vi "Capacitance_IS_Configure.vi"(0 "Semiconductor Module Context":T7, 1 "DCPower Pin":tag, 2 "Scope Pins":tag[](array[tag]), 3 "FGEN Pin":tag, 4 "SCOPE Parameters":T4={"min sample rate"=20000000.0, "min record length"=1000, "reference position"=5.0, "input impedance"=0, "maximum input frequency"=0.0, "vertical coupling"=1, "vertical range"=10.0, "vertical offset"=0.0, "NumRecords"=0} {"maximum input frequency" format="%.2f"; "input impedance" items=["1 mega ohm"=0, "50 ohms"=2]; "vertical offset" format="%.4f"; "vertical range" format="%.2f"; "vertical coupling" items=["AC", "DC", "Ground"]; "reference position" format="%#_13g"; "min sample rate" format="%^.2e"}, 5 "FGEN Parameters":T2 {"Trigger Mode" items=["Single", "Continuous", "Stepped", "Burst"]}, 6 "DCPower_Parameters":T6={"Output"=enum."DC Voltage", "Current_range"=0.0, "Current"=0.0, "Voltage_range"=0.0, "Voltage"=0.0, "Aperture_time"=0.0, "Source Delay"=0.0, "Sense"=1008} {"Source Delay" format="%.6p"; "Sense" items=["Local"=1008, "Remote"=1009]; "Aperture_time" format="%.6p"; "Current_range" format="%.6p"; "Current" format="%.6p"; "Voltage_range" format="%.6p"; "Voltage" format="%.6p"}) -> (14 "FFT Subset Parameters":T1, 19 "error out":errorcluster)   [LabVIEW 2023, in "Capacitance.lvlib"]
doc: "Configure DCPower, SCOPE and FGEN sessions for impedance spectroscopy measurement"
uses:
  Capacitance.lvlib
  <vilib>/NI_TestStand_SemiconductorModule/NI_TestStand_Semiconductor_Module.lvlibp/PinMap/General/SemiconductorModuleContext.ctl
  ResourceHandling/TypeDefs/RH_DCPower_Parameters.ctl
  ResourceHandling/TypeDefs/RH_SCOPE_Parameters.ctl
  <instrlib>/niScope/Controls/niScope vertical coupling.ctl
  ResourceHandling/TypeDefs/RH_FGEN_Parameters.ctl
  <instrlib>/niFgen/niFgen.llb/niFgen Trigger Mode.ctl
  <instrlib>/niFgen/niFgen.llb/niFgen_ctl Exported Signal Desination Values (ComboBox).ctl
  <instrlib>/niScope/Controls/niScope trigger source digital.ctl
  <vilib>/NI_TestStand_SemiconductorModule/NI_TestStand_Semiconductor_Module.lvlibp/PinMap/DC Power/PinToNIDCPowerSessions.vi
  <vilib>/NI_TestStand_SemiconductorModule/NI_TestStand_Semiconductor_Module.lvlibp/PinMap/Scope/PinsToNISCOPESession.vi
  <vilib>/NI_TestStand_SemiconductorModule/NI_TestStand_Semiconductor_Module.lvlibp/PinMap/FGEN/PinToNIFGenSession.vi
  <vilib>/NI_TestStand_SemiconductorModule/NI_TestStand_Semiconductor_Module.lvlibp
  ResourceHandling/ResourceHandling.lvlib
  Resonance/Resonance.lvlib
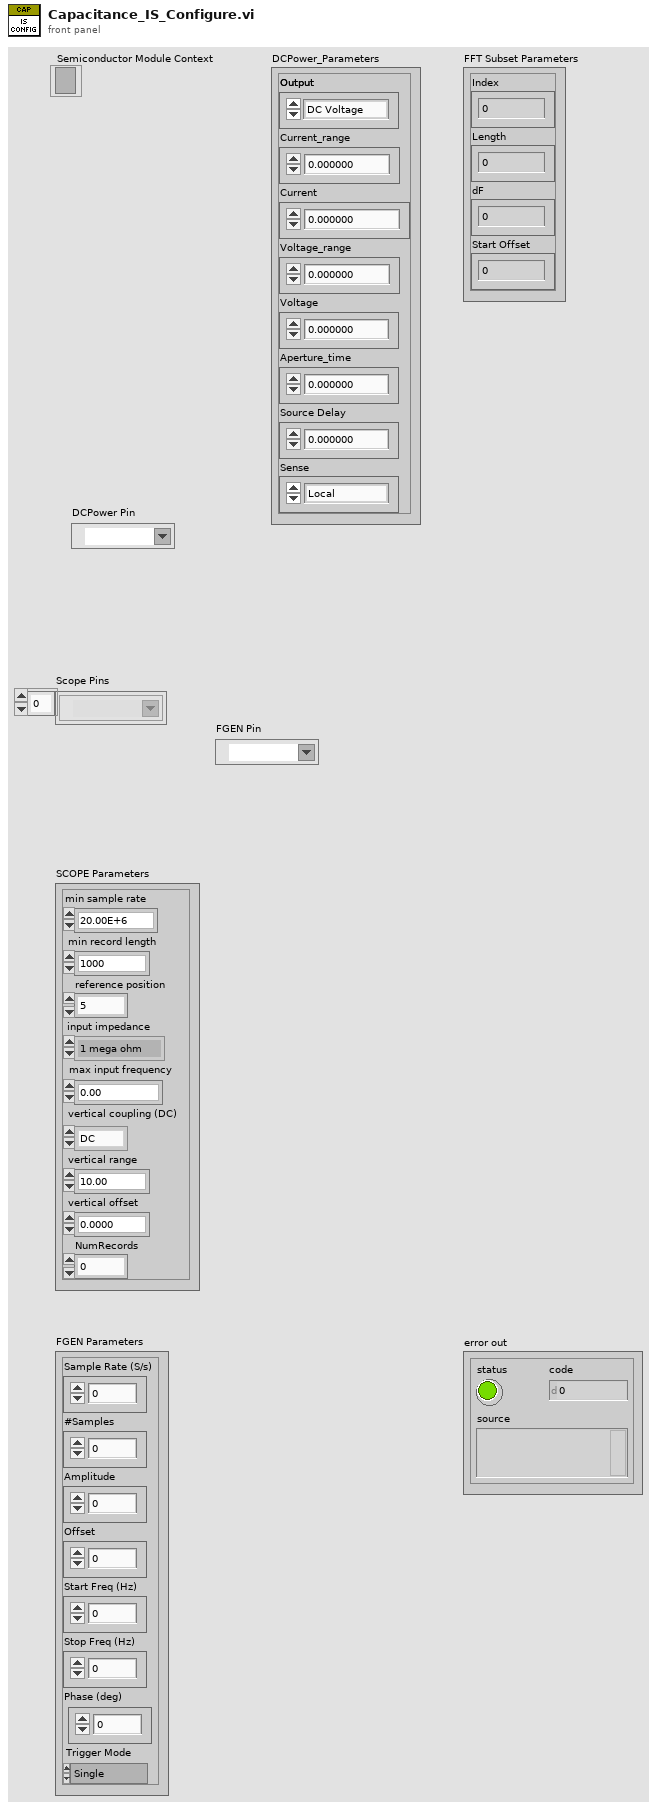
[diagram p1: front panel]
types:
  T1 = cluster{"Index":i32, "Length":i32, "dF":dbl, "Start Offset":dbl}
  T2 = typedef "ResourceHandling.lvlib/RH_FGEN_Parameters.ctl" = cluster{"Sample Rate (S/s)":dbl, "#Samples":i32, "Amplitude":dbl, "Offset":dbl, "Start Freq (Hz)":dbl, "Stop Freq (Hz)":dbl, "Phase (deg)":dbl, "Trigger Mode":T3}
  T3 = typedef "niFgen Trigger Mode.ctl" = i32
  T4 = typedef "ResourceHandling.lvlib/RH_SCOPE_Parameters.ctl" = cluster{"min sample rate":dbl, "min record length":i32, "reference position":dbl, "input impedance":u32, "maximum input frequency":dbl, "vertical coupling":T5, "vertical range":dbl, "vertical offset":dbl, "NumRecords":i32}
  T5 = typedef "niScope vertical coupling.ctl" = i32
  T6 = typedef "ResourceHandling.lvlib/RH_DCPower_Parameters.ctl" = cluster{"Output":enum16{"DC Voltage", "DC Current"}, "Current_range":dbl, "Current":dbl, "Voltage_range":dbl, "Voltage":dbl, "Aperture_time":dbl, "Source Delay":dbl, "Sense":i32}
  T7 = typedef "NI_TestStand_Semiconductor_Module.lvlibp/SemiconductorModuleContext.ctl" = refnum<k7>
  T8 = typedef "niScope trigger source digital.ctl" = string
  T9 = typedef "niFgen_ctl Exported Signal Desination Values (ComboBox).ctl" = string
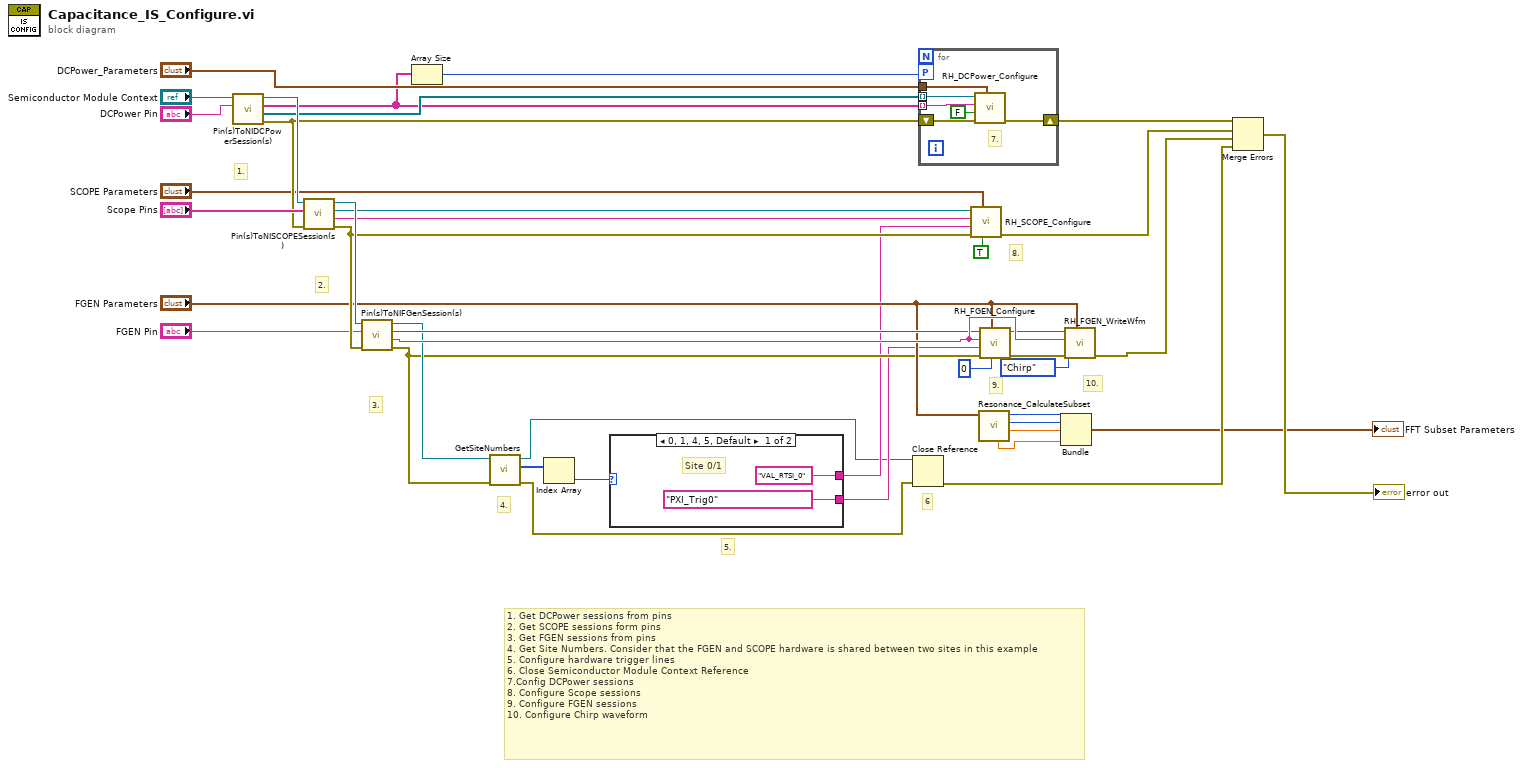
[diagram p0: block diagram]
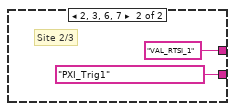
[diagram p2: hidden frame]
diagram:
  # "5."
  # "4."
  # "8."
  # "10."
  # "9."
  # "1. Get DCPower sessions from pins\n2. Get SCOPE sessions form pins\n3. Get FGEN sessions from pins\n4. Get Site Numbers. Consider that the FGEN and SCOPE hardware is shared between two sites in this example\n5. Configure hardware trigger lines \n6. Close Semiconductor Module Context Reference\n7.Config DCPower sessions\n8. Configure Scope sessions\n9. Configure FGEN sessions \n10. Configure Chirp waveform"
  # "6"
  # "3."
  # "2."
  # "1."
  n1 = call-poly <vilib>:"Pin(s)ToNIDCPowerSession(s).vi"("Pin"="DCPower Pin", "Semiconductor Module Context"="Semiconductor Module Context") -> ("error out"=w38:errorcluster, "Instrument Sessions"=w27:refnum<k15>[], "Channel Strings"=w9:string[], "Semiconductor Module Context Out"=w39:T7)  [unwired: 5 in, 1 out]
  n2 = call-poly <vilib>:"Pin(s)ToNISCOPESession(s).vi"("error in (no error)"=w38, "Pins"="Scope Pins", "Semiconductor Module Context"=w39) -> ("error out"=w30:errorcluster, "Channel List"=w31:string, "Instrument Session"=w26:refnum<k15>, "Semiconductor Module Context Out"=w35:T7)  [unwired: 4 in, 1 out]
  n3 = call-poly <vilib>:"Pin(s)ToNIFGenSession(s).vi"("error in (no error)"=w30, "Pin"="FGEN Pin", "Semiconductor Module Context"=w35) -> ("error out"=w7:errorcluster, "Channel List"=w28:string, "Instrument Session"=w25:refnum<k15>, "Semiconductor Module Context Out"=w8:T7)  [unwired: 4 in, 1 out]
  n4 = Array Size(array=w9) -> (size(s)=w10:i32)
  n5 = call <vilib>:"GetSiteNumbers.vi"("error in (no error)"=w7, "Semiconductor Module Context"=w8) -> ("error out"=w1:errorcluster, "Site Numbers"=w6:i32[], "Semiconductor Module Context Out"=w2:T7)  [unwired: 6 in, 1 out]
  n6 = Index Array(array=w6) -> (element=w5:i32)  [unwired: 1 in]
  n7 = case shown="0, 1, 4, 5, Default" w5 {
    tunnel: [T9 "PXI_Trig0" ("Output Terminal (do not export)") T9 "PXI_Trig1" ("Output Terminal (do not export)")] -> w4
    tunnel: [T8 "VAL_RTSI_0" ("trigger source") T8 "VAL_RTSI_1" ("trigger source")] -> w3
    frame 0, 1, 4, 5, Default {
      # "Site 0/1"
    }
    frame 2, 3, 6, 7 {
      # "Site 2/3"
    }
  }
  n8 = Close Reference(reference=w2, error in (no error)=w1) -> (error out=w36:errorcluster)
  n9 = for {
    tunnel: w9 -> [w50] mode=indexing
    tunnel: "DCPower_Parameters" -> [w48]
    tunnel: w27 -> [w47] mode=indexing
    shift-right: [w49] -> w37
    shift-left: w38 -> [w51]
    workers-P: w10 -> [_]
    # "7."
    n10 = call "RH_DCPower_Configure.vi"("DCPower_Parameters"=w48, "error in (no error)"=w51, "trigger out?"=FALSE, "channel name"=w50, "DCPower Session In"=w47) -> ("error out"=w49:errorcluster)  [unwired: 5 in, 1 out]
  }
  n11 = call "RH_SCOPE_Configure.vi"("Digital Trigger?"=TRUE, "SCOPE Global Parameters"="SCOPE Parameters", "error in"=w30, "trigger source"=w3, "channels"=w31, "SCOPE Session In"=w26) -> ("error out"=w29:errorcluster)  [unwired: 4 in, 1 out]
  n12 = call "Resonance_CalculateSubset.vi"("FGEN Parameters"="FGEN Parameters") -> ("dF"=w20:dbl, "Length"=w21:i32, "Index"=w22:i32, "Start Offset"=w19:dbl)  [unwired: 6 in, 1 out]
  n13 = call "RH_FGEN_Configure.vi"("Marker Position"=0, "FGEN Parameters"="FGEN Parameters", "error in"=w7, "Output Terminal (do not export)"=w4, "Channel Name"=w28, "FGEN Session In"=w25) -> ("error out"=w16:errorcluster, "FGEN Session Out"=w15:refnum<k15>)  [unwired: 4 in]
  n14 = Bundle("Index"=w22, "Length"=w21, "dF"=w20, "Start Offset"=w19) -> (→"FFT Subset Parameters":T1)  [unwired: 1 in]
  n15 = call "RH_FGEN_WriteWfm.vi"("FGEN Parameters"="FGEN Parameters", "error IO"=w16, "Wfm Type"=enum16{"Chirp", "MultiSine", "Sine"}."Chirp", "Channel Name"=w28, "FGEN Session In"=w15) -> ("error out"=w24:errorcluster)  [unwired: 5 in, 1 out]
  n16 = Merge Errors(w37, w29, w24, w36) -> (→"error out":errorcluster)
